vi "Get_Access_Token.vi"(8 "error in (no error)":errorcluster, 11 "OneNote in":refnum<class "OneNote.lvclass">) -> (0 "error out":errorcluster, 2 "Access Token":string, 3 "OneNote out":refnum<class "OneNote.lvclass">)   [LabVIEW 2016, in "OneNote.lvclass"]
uses:
  OneNote.lvclass
  OneNote.lvclass/OneNote.ctl
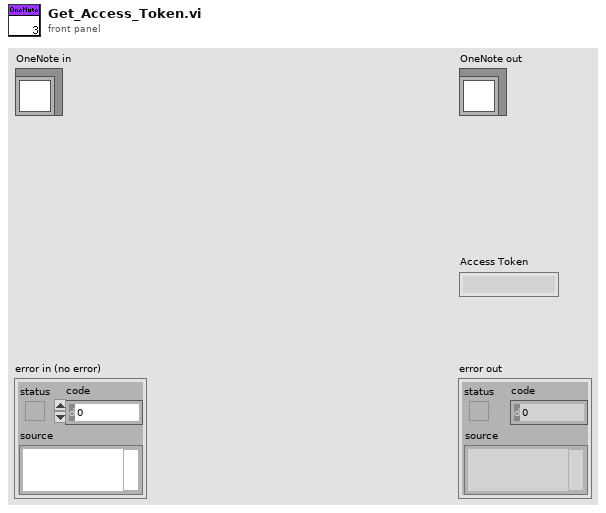
[diagram p1: front panel]
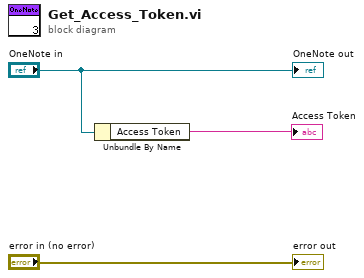
[diagram p0: block diagram]
diagram:
  n1 = Unbundle By Name("OneNote in") -> ("Access Token"=→"Access Token":string)
  "error out" <- "error in (no error)"
  "OneNote out" <- "OneNote in"
